vi "gc-zyklus mfc mpos konfig.vi"() -> ()   [LabVIEW 2010]
uses:
  <vilib>/Instr/_visa.llb/VISA Configure Serial Port (Instr).vi
panel:
  in  "Notabschaltung":bool=TRUE
  in  "Konfigurationsdatei auswählen":path
  out "Konfiguration":string
  out "Zeitpunkt":string
  out "Temperatur (°C)":u16
  out "Meßwert PC2 (mbara)":u16
  out "Meßwert PC1 (mbara)":u16
  out "Meßwert FC (mln/min)":u16
  in  "Setpoint PC1 (bara)":dbl min=0.15 max=3.0 step=0.05
  in  "Setpoint PC2 (bara)":dbl min=0.15 max=3.0 step=0.05
  in  "Messwerte speichern":path
  out "Zyklus Nr.":i32
  out "Positionen (1-6)":i32[](array[numeric])=[1, 3, 5, 2]
  out "Anzahl der Zustände (Mpos.-Ventil)":i32
  out "aktuelle Position":i32
  out "Setpoints FC (ln/min)":dbl[](array[numeric])=[1.0, 3.0, 5.0, 2.0]
  out "Längen der Zustände (s)":i32[](array[numeric])=[1, 3, 5, 2]
  out "Anzahl der Zustände (MFC)":i32
  out "Länge des aktuellen Zustandes (s)":i32
  out "aktueller Setpoint FC (ln/min)":dbl
  out "Sequenz Nr.":i32
  out "Aktuelle Zeit":timestamp
  in  "(Sequenz wird gesittet zu Ende geführt)":bool
  # "Gerät im Chromatographie-Zyklus, z.B. MFC"
  # "Multipositionsventil"
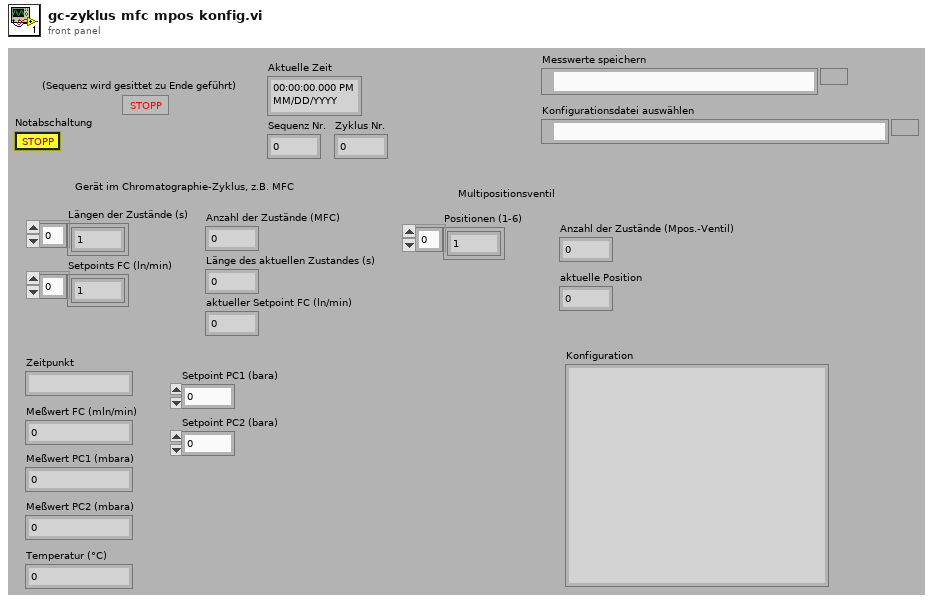
[diagram p1: front panel]
types:
  T1 = enum16{"open", "replace", "create", "open or create", "replace or create", "replace or create with confirmation"}
  T2 = cluster{"Mode":enum16{"RTU", "ASCII"}, "Slave Address":u8}
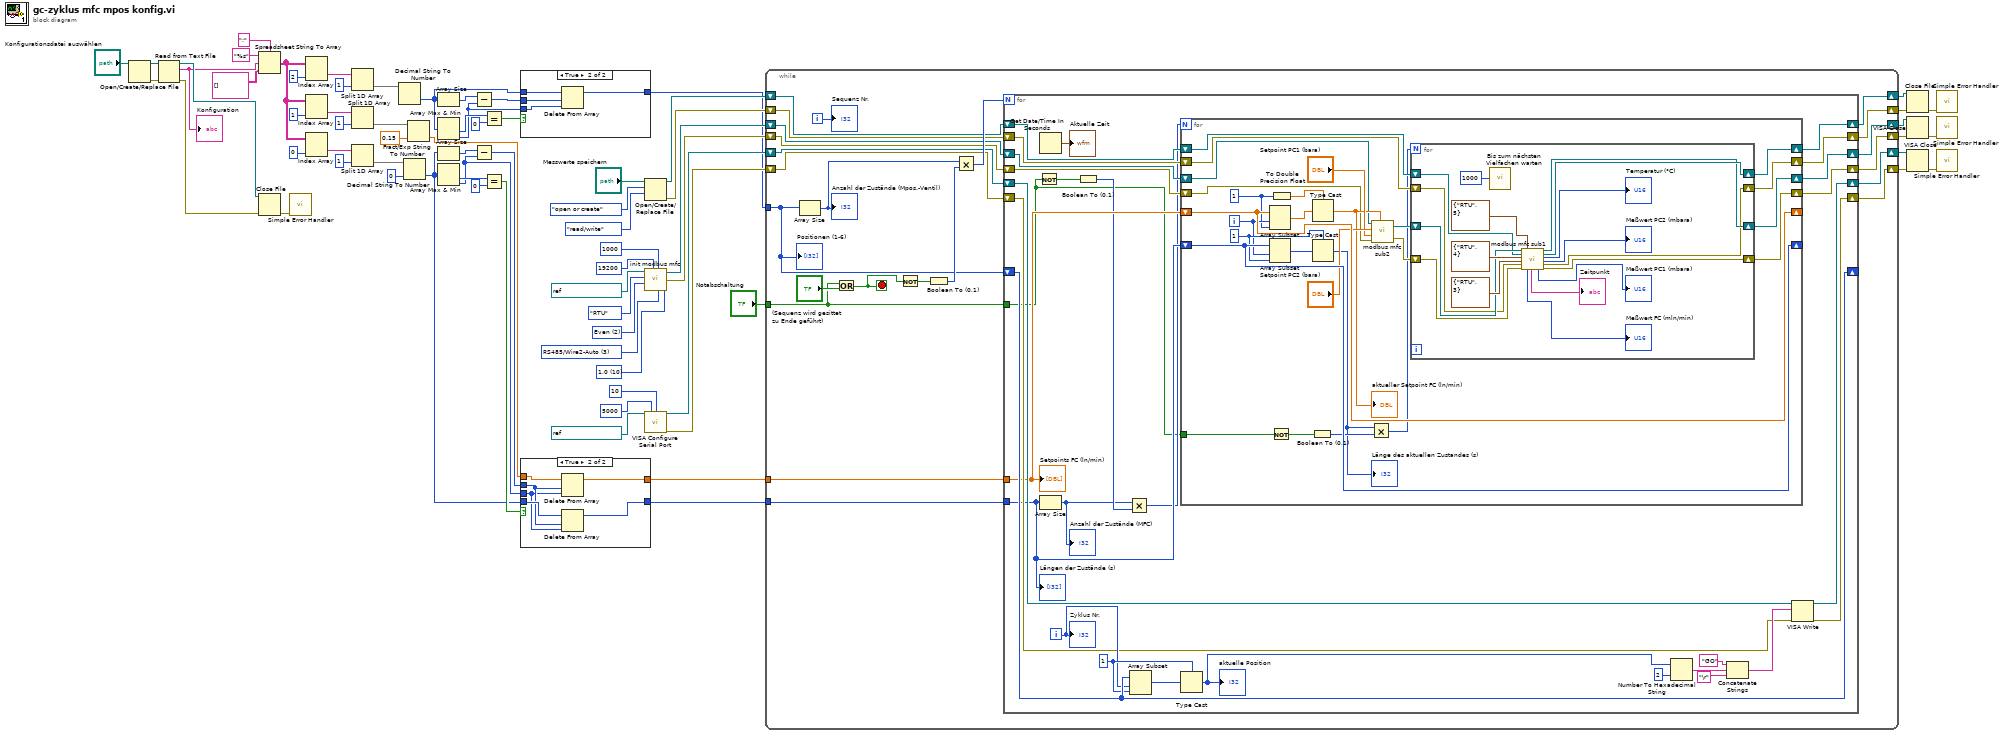
[diagram p0: block diagram]
diagram:
  w69 = u16 10 items=["1.0"=10, "1.5"=15, "2.0"=20] ("Serial Settings:Stop Bits")
  w67 = u16 2 items=["None", "Odd", "Even", "Mark", "Space"] ("Parity")
  w68 = i16 3 items=["Unknown"=-1, "RS485/Wire4"=0, "RS485/Wire2-EchoDTR"=1, "RS485/Wire2-CtrlDTR"=2, "RS485/Wire2-Auto"=3, "RS232/DTE"=128, "RS232/DCE"=129, "RS232/AUTO"=130] ("Serial Settings:Wire Mode")
  n1 = Open/Create/Replace File(file path (use dialog)="Konfigurationsdatei auswählen") -> (refnum out=w44:refnum<file>, error out=w43:errorcluster)  [unwired: 5 in, 1 out]
  n2 = Read from Text File(file (use dialog)=w44, error in=w43) -> (refnum out=w41:refnum<file>, text=w38:string, error out=w42:errorcluster)  [unwired: 2 in, 1 out]
  "Konfiguration" <- w38
  n3 = Spreadsheet String To Array(delimiter (Tab)=";", format string="%s" ("Format-String"), spreadsheet string=w38, array type (2D Dbl)=string[][] []) -> (array=w10:string[][])
  n4 = Close File(refnum=w41, error in=w42) -> (error out=w40:errorcluster)  [unwired: 1 out]
  n5 = call <vilib>:"Simple Error Handler.vi"("error in (no error)"=w40) -> ()  [unwired: 4 in, 5 out]
  n6 = Index Array(array=w10, index (col)=2 ("Index")) -> (element=w22:string[])  [unwired: 1 in]
  n7 = Index Array(array=w10, index (col)=1 ("Index")) -> (element=w16:string[])  [unwired: 1 in]
  n8 = Index Array(array=w10, index (col)=0 ("Index")) -> (element=w12:string[])  [unwired: 1 in]
  n9 = Split 1D Array(array=w22, index=1 ("Index")) -> (second subarray=w20:string[])  [unwired: 1 out]
  n10 = Split 1D Array(array=w16, index=1 ("Index")) -> (second subarray=w14:string[])  [unwired: 1 out]
  n11 = Split 1D Array(array=w12, index=1 ("Index")) -> (second subarray=w7:string[])  [unwired: 1 out]
  n12 = Decimal String To Number(string=w20) -> (number=w24:i32[])  [unwired: 2 in, 1 out]
  n13 = Decimal String To Number(string=w7, default (0L)=0 ("Standard (0 I32)")) -> (number=w26:i32[])  [unwired: 1 in, 1 out]
  n14 = Fract/Exp String To Number(string=w14, default (0 dbl)=0.15 ("Standard (0 DBL)")) -> (number=w25:dbl[])  [unwired: 2 in, 1 out]
  n15 = Array Size(array=w24) -> (size(s)=w19:i32)
  n16 = Array Max & Min(array=w24) -> (min value=w34:i32, min index (indices)=w18:i32)  [unwired: 2 out]
  n17 = Array Size(array=w26) -> (size(s)=w9:i32)
  n18 = Array Max & Min(array=w26) -> (min value=w30:i32, min index (indices)=w8:i32)  [unwired: 2 out]
  n19 = Subtract(x=w19, y=w18) -> (x-y=w31:i32)
  n20 = Subtract(x=w9, y=w8) -> (x-y=w27:i32)
  n21 = Equal?(x=w34, y=0) -> (x = y?=w32:bool)
  n22 = Equal?(x=w30, y=0) -> (x = y?=w28:bool)
  n23 = case shown="True" w32 {
    tunnel: w24 -> [w73 w77]
    tunnel: w18 -> [_ w75]
    tunnel: [w73 w76] -> w6
    tunnel: w31 -> [_ w74]
    frame False {
    }
    frame True {
      n24 = Delete From Array(array=w77, length=w74, index=w75) -> (array with subset deleted=w76:i32[])  [unwired: 1 out]
    }
  }
  n25 = case shown="True" w28 {
    tunnel: w26 -> [w79 w85]
    tunnel: w8 -> [_ w80]
    tunnel: [w79 w84] -> w4
    tunnel: w27 -> [_ w81]
    tunnel: w25 -> [w78 w83]
    tunnel: [w78 w82] -> w5
    frame False {
    }
    frame True {
      n26 = Delete From Array(array=w83, length=w81, index=w80) -> (array with subset deleted=w82:dbl[])  [unwired: 1 out]
      n27 = Delete From Array(array=w85, length=w81, index=w80) -> (array with subset deleted=w84:i32[])  [unwired: 1 out]
    }
  }
  n28 = Open/Create/Replace File(file path (use dialog)="Messwerte speichern", operation (0:open)=T1."open or create" ("Operation (0:Öffnen)"), access (0:read/write)=enum16{"read/write", "read-only", "write-only"}."read/write" ("Zugriff (0:Lesen/Schreiben)")) -> (refnum out=w62:refnum<file>, error out=w61:errorcluster)  [unwired: 3 in, 1 out]
  n29 = call "init modbus mfc.vi"("Timeout"=u32 1000, "Serial Settings:Stop Bits"=w69, "Serial Settings:Wire Mode"=w68, "Baud Rate"=u32 19200, "VISA resource name"=refnum<visa-resource-name> "ASRL2::INSTR", "Mode"=enum16{"RTU", "ASCII"}."RTU", "Parity"=w67) -> ("VISA resource name out"=w60:refnum<visa-resource-name>, "error out"=w59:errorcluster)  [unwired: 2 in]
  n30 = call-poly "VISA Configure Serial Port"("VISA resource name"=refnum<visa-resource-name> "ASRL1::INSTR", "timeout (10sec)"=u32 5000, "termination char\n(0xA = '\\n' = LF)"=u8 10 ("termination char\n(0xA = '\\n' = LF)")) -> ("VISA resource name out"=w49:refnum<visa-resource-name>, "error out"=w48:errorcluster)  [unwired: 11 in]
  n31 = while {
    shift-right: [w99] -> w53
    shift-left: w62 -> [w103]
    shift-right: [w98] -> w52
    shift-left: w61 -> [w102]
    shift-right: [w97] -> w51
    shift-left: w60 -> [w101]
    shift-right: [w96] -> w50
    shift-left: w59 -> [w100]
    shift-right: [w93] -> w46
    shift-left: w49 -> [w95]
    shift-right: [w92] -> w45
    shift-left: w48 -> [w94]
    tunnel: w6 -> [w91]
    tunnel: w5 -> [w90]
    tunnel: w4 -> [w89]
    tunnel: "Notabschaltung" -> [w86]
    i -> [w108]
    stop <- w88 stop-if-true
    n32 = Array Size(array=w91) -> (size(s)=w107:i32)
    "Anzahl der Zustände (Mpos.-Ventil)" <- w107
    n33 = Or(x=w86, y="(Sequenz wird gesittet zu Ende geführt)") -> (x .or. y?=w88:bool)
    n34 = Not(x=w88) -> (.not. x?=w106:bool)
    n35 = Boolean To (0,1)(Boolean=w106) -> (0, 1=w104:i16)
    n36 = Multiply(x=w107, y=w104) -> (x*y=w105:i32)
    n37 = for {
      N: w105 -> [_]
      shift-right: [w138] -> _
      shift-left: w91 -> [w138]
      shift-right: [w123] -> w99
      shift-left: w103 -> [w130]
      shift-right: [w122] -> w98
      shift-left: w102 -> [w131]
      shift-right: [w121] -> w97
      shift-left: w101 -> [w133]
      shift-right: [w120] -> w96
      shift-left: w100 -> [w132]
      shift-right: [w117] -> w93
      shift-left: w95 -> [w119]
      shift-right: [w116] -> w92
      shift-left: w94 -> [w118]
      tunnel: w90 -> [w115]
      tunnel: w89 -> [w114]
      tunnel: w86 -> [w109]
      i -> [w135]
      w137 = 1 ("Länge")
      n38 = Not(x=w109) -> (.not. x?=w113:bool)
      n39 = Get Date/Time In Seconds() -> (seconds since 1Jan1904=→"Aktuelle Zeit":timestamp)
      n40 = Array Size(array=w114) -> (size(s)=w111:i32)
      "Anzahl der Zustände (MFC)" <- w111
      n41 = Boolean To (0,1)(Boolean=w113) -> (0, 1=w112:i16)
      n42 = Multiply(x=w111, y=w112) -> (x*y=w110:i32)
      n43 = Array Subset(array=w138, index=w135, length=w137) -> (w136:i32[])
      n44 = for {
        N: w110 -> [_]
        shift-right: [w164] -> _
        shift-left: w114 -> [w164]
        shift-right: [w160] -> _
        shift-left: w115 -> [w160]
        shift-right: [w154] -> w123
        shift-left: w130 -> [w155]
        shift-right: [w152] -> w122
        shift-left: w131 -> [w156]
        shift-right: [w153] -> w121
        shift-left: w133 -> [w147]
        shift-right: [w151] -> w120
        shift-left: w132 -> [w146]
        tunnel: w109 -> [w141]
        i -> [w159]
        w158 = 1 ("Länge")
        w163 = 1 ("Länge")
        n45 = Array Subset(array=w160, index=w159, length=w158) -> (w161:dbl[])
        n46 = Array Subset(array=w164, index=w159, length=w163) -> (w162:i32[])
        n47 = Not(x=w141) -> (.not. x?=w143:bool)
        n48 = To Double Precision Float(number=w158) -> (double precision float=w157:dbl)
        n49 = Boolean To (0,1)(Boolean=w143) -> (0, 1=w142:i16)
        n50 = Type Cast(type=w157, x=w161) -> (*(type *) &x=w148:dbl)
        "aktueller Setpoint FC (ln/min)" <- w148
        n51 = Type Cast(type=w163, x=w162) -> (*(type *) &x=w140:i32)
        "Länge des aktuellen Zustandes (s)" <- w140
        n52 = Multiply(x=w140, y=w142) -> (x*y=w139:i32)
        n53 = call "modbus mfc sub2.vi"("VISA resource name out 2"=w147, "Setpoint PC2 (bara)"="Setpoint PC2 (bara)", "Setpoint PC1 (bara)"="Setpoint PC1 (bara)", "error out 2"=w146, "Setpoint FC (ln/min)"=w148) -> ("VISA resource name out"=w145:refnum<visa-resource-name>, "error out"=w144:errorcluster)
        n54 = for {
          N: w139 -> [_]
          shift-right: [w167] -> w153
          shift-left: w145 -> [w171]
          shift-right: [w168] -> w154
          shift-left: w155 -> [w169]
          shift-right: [w166] -> w152
          shift-left: w156 -> [w170]
          shift-right: [w165] -> w151
          shift-left: w144 -> [w172]
          n55 = call "Bis zum nächsten Vielfachen warten"("Count(mSec)"=u32 1000) -> ()  [unwired: 1 out]
          n56 = call "modbus mfc sub1.vi"("VISA resource name out"=w171, "refnum out 2"=w169, "Serial Parameters 2"=T2 {"Mode"=enum."RTU", "Slave Address"=4}, "Serial Parameters"=T2 {"Mode"=enum."RTU", "Slave Address"=3}, "error out 2"=w170, "error out 3"=w172, "Serial Parameters 3"=T2 {"Mode"=enum."RTU", "Slave Address"=5}) -> ("Numerisch 3"=→"Meßwert FC (mln/min)":u16, "date/time string"=→"Zeitpunkt":string, "Numerisch 2"=→"Meßwert PC1 (mbara)":u16, "VISA resource name out 2"=w167:refnum<visa-resource-name>, "refnum out"=w168:refnum<file>, "Numerisch 4"=→"Temperatur (°C)":u16, "Numerisch"=→"Meßwert PC2 (mbara)":u16, "error out"=w166:errorcluster, "error out 4"=w165:errorcluster)  [unwired: 3 in, 1 out]
        }
      }
      n57 = Type Cast(type=w137, x=w136) -> (*(type *) &x=w124:i32)
      "aktuelle Position" <- w124
      n58 = Number To Hexadecimal String(1:i16 2 ("Breite (-)"), 2:w124) -> (0:w128:string)
      n59 = Concatenate Strings("GO" ("String"), w128, "\r") -> (w129:string)
      n60 = VISA Write(VISA resource name=w119, write buffer=w129, error in (no error)=w118) -> (VISA resource name out=w117:refnum<visa-resource-name>, error out=w116:errorcluster)  [unwired: 1 out]
      "Längen der Zustände (s)" <- w114
      "Setpoints FC (ln/min)" <- w115
      "Zyklus Nr." <- w135
    }
    "Positionen (1-6)" <- w91
    "Sequenz Nr." <- w108
  }
  n61 = Close File(refnum=w53, error in=w52) -> (error out=w57:errorcluster)  [unwired: 1 out]
  n62 = VISA Close(VISA resource name=w51, error in (no error)=w50) -> (error out=w58:errorcluster)
  n63 = VISA Close(VISA resource name=w46, error in (no error)=w45) -> (error out=w47:errorcluster)
  n64 = call <vilib>:"Simple Error Handler.vi"("error in (no error)"=w57) -> ()  [unwired: 4 in, 5 out]
  n65 = call <vilib>:"Simple Error Handler.vi"("error in (no error)"=w58) -> ()  [unwired: 4 in, 5 out]
  n66 = call <vilib>:"Simple Error Handler.vi"("error in (no error)"=w47) -> ()  [unwired: 4 in, 5 out]
